vi "IsLaserReady.vi"(3 "error in":errorcluster) -> (0 "error out":errorcluster, 2 "Ready?":bool)   [LabVIEW 2012]
uses:
  bin/OVA32.dll
panel:
  out "DLL Return Code":i32
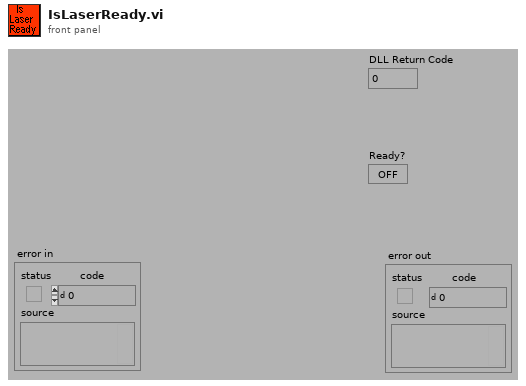
[diagram p1: front panel]
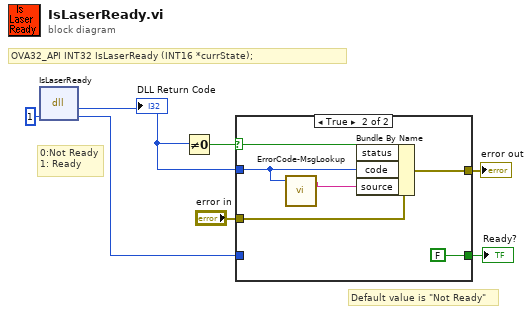
[diagram p0: block diagram]
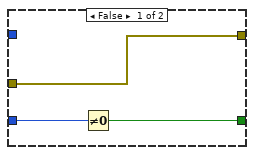
[diagram p2: hidden frame]
diagram:
  # "OVA32_API INT32 IsLaserReady (INT16 *currState);"
  # "Default value is \"Not Ready\""
  # "0:Not Ready\n1: Ready"
  n1 = dll-call lib="C:/_src/OVA5000_DSP_falcon/Software/LabVIEW/OVA/SDK/OVA_5000_SDK_v5.14.3/bin/OVA32.dll" fn="IsLaserReady"("currState"=i16 1) -> (w5:i32, "currState"=w2:i16)  [unwired: 3 in, 2 out]
  "DLL Return Code" <- w5
  n2 = Not Equal To 0?(x=w5) -> (x != 0?=w6:bool)
  n3 = case shown="True" w6 {
    selector: w6 -> [_ w13]
    tunnel: w5 -> [_ w12]
    tunnel: "error in" -> [w10 w15]
    tunnel: [w10 w14] -> w4
    tunnel: w2 -> [w9 _]
    tunnel: [w8 FALSE] -> w3
    frame False {
      n4 = Not Equal To 0?(x=w9) -> (x != 0?=w8:bool)
    }
    frame True {
      n5 = call "ErrorCode-MsgLookup.vi"("DLL Return Code"=w12) -> ("Error String"=w16:string)  [unwired: 2 in, 2 out]
      n6 = Bundle By Name(cluster=w15, "status"=w13, "code"=w12, "source"=w16) -> (w14:errorcluster)
    }
  }
  "Ready?" <- w3
  "error out" <- w4
